vi "Write Inverted.vi"(8 "error in (no error)":errorcluster, 10 "Inverted?":bool, 11 "Switch in":refnum<class "Switch.lvclass">) -> (0 "error out":errorcluster, 3 "Switch out":refnum<class "Switch.lvclass">)   [LabVIEW 2016, in "Switch.lvclass"]
uses:
  Switch.lvclass
  Switch.lvclass/Switch.ctl
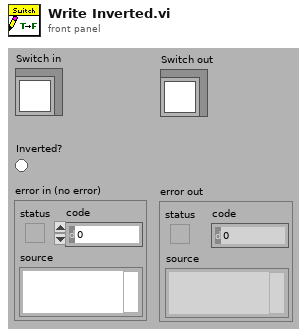
[diagram p1: front panel]
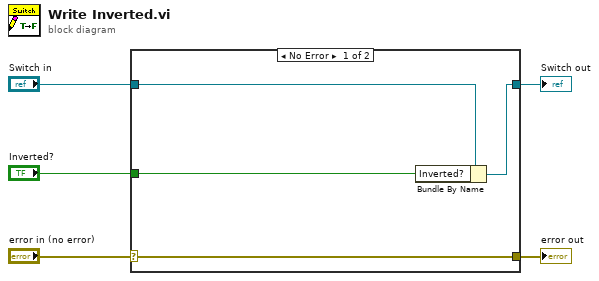
[diagram p0: block diagram]
diagram:
  n1 = case shown="No Error" "error in (no error)" {
    selector: "error in (no error)" -> [w9 w10]
    tunnel: [w9 w10] -> w4
    tunnel: [w7 w11] -> w2
    tunnel: "Switch in" -> [w8 w11]
    tunnel: "Inverted?" -> [w6 _]
    frame No Error {
      n2 = Bundle By Name(cluster=w8, "Inverted?"=w6) -> (w7:refnum<class "Switch.lvclass">)
    }
    frame Error {
    }
  }
  "error out" <- w4
  "Switch out" <- w2
